vi "4Pi 4Pi Modes - Init DM DUAL.vi"(8 "No hardware":bool=TRUE, 9 "Config File":string, 11 "Base File Path":path) -> (2 "Error out":errorcluster, 3 "DM Handles":T1(array[cluster]))   [LabVIEW 2016]
uses:
  4Pi 4Pi Modes - Controls/4Pi 4Pi Modes - Standard Action.ctl
  Hardware Configuration/Hardware Configuration Controls/Standard Action.ctl
  <userlib>/BMC/BMC.lvlib
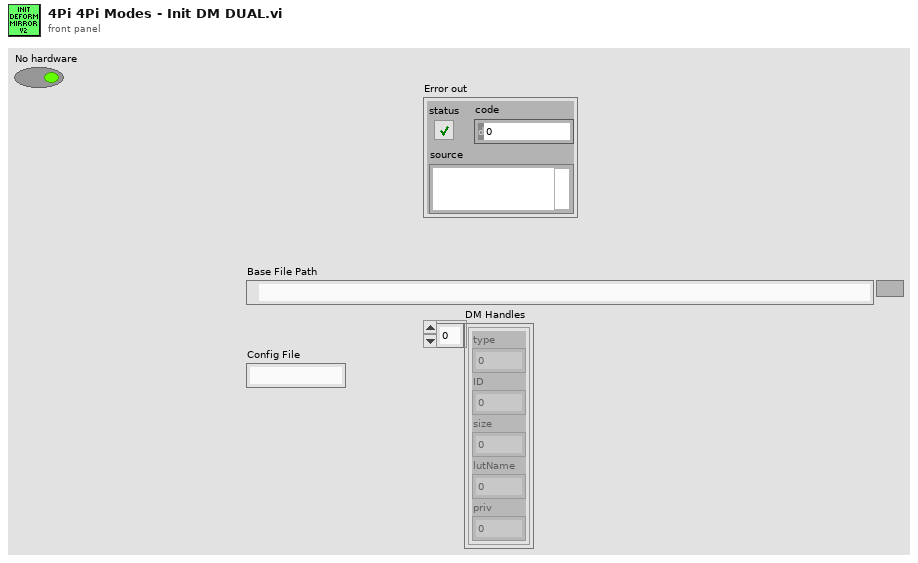
[diagram p1: front panel]
types:
  T1 = cluster{"type":i16, "ID":i16, "size":i32, "lutName":u64, "priv":u64}[]
  T2 = typedef "Standard Action.ctl" = enum16{"Read", "Write"}
  T3 = typedef "4Pi 4Pi Modes - Standard Action.ctl" = enum16{"Read", "Write"}
  T4 = cluster{"Matrix":dbl[][], "Modes":string[], "Flats":dbl[], "Serials":string[]}
  T5 = cluster{"type":i16, "ID":i16, "size":i32, "lutName":u64, "priv":u64}
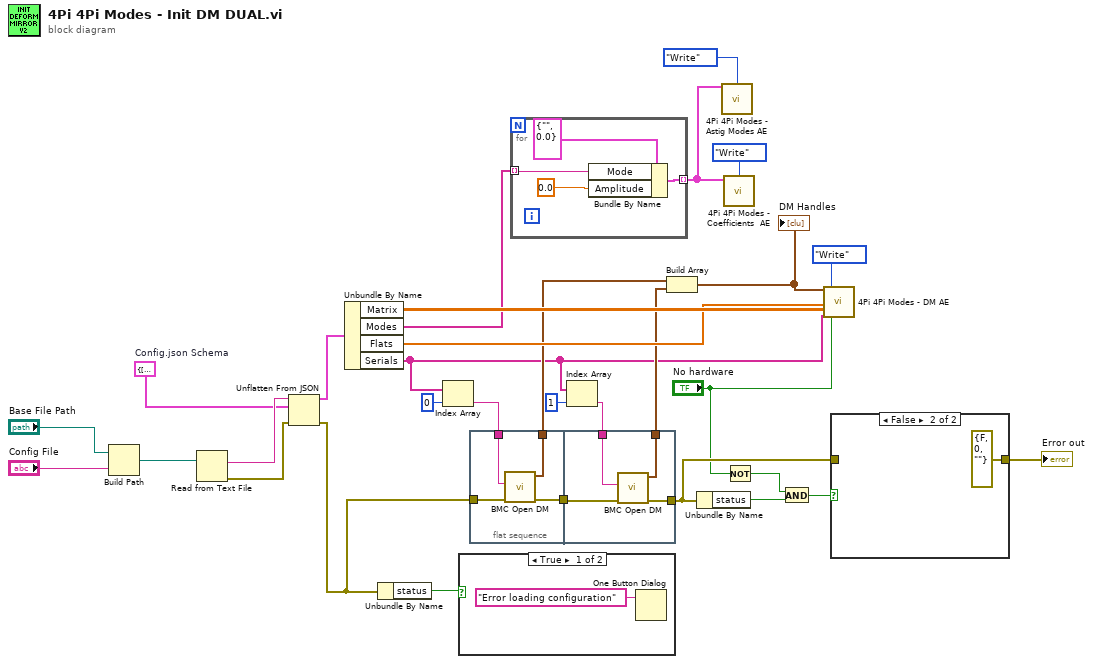
[diagram p0: block diagram]
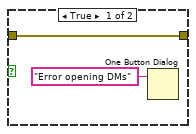
[diagram p2: hidden frame]
diagram:
  w25 = T4 {"Matrix"=[], "Modes"=[], "Flats"=[], "Serials"=[]}  # Config.json Schema
  n1 = Build Path(base path="Base File Path", name or relative path="Config File") -> (appended path=w28:path)
  n2 = Read from Text File(file (use dialog)=w28) -> (text=w26:string, error out=w19:errorcluster)  [unwired: 3 in, 2 out]
  n3 = Unflatten From JSON(JSON string=w26, type and defaults=w25, error in (no error)=w19) -> (value=w24:T4, error out=w18:errorcluster)  [unwired: 4 in]
  n4 = Unbundle By Name(w24) -> ("Matrix"=w23:dbl[][], "Modes"=w9:string[], "Flats"=w22:dbl[], "Serials"=w2:string[])
  n5 = Unbundle By Name(w18) -> ("status"=w27:bool)
  n6 = Index Array(array=w2, index=0) -> (element=w13:string)
  n7 = case shown="True" w27 {
    frame True {
      n8 = One Button Dialog(message="Error loading configuration") -> ()  [unwired: 1 in, 1 out]
    }
    frame False {
    }
  }
  n9 = flat-sequence {
    tunnel: [w36] -> w20
    tunnel: [w35] -> w17
    tunnel: w18 -> [w34]
    tunnel: w13 -> [w33]
    tunnel: w20 -> [w40]
    tunnel: [w39] -> w16
    tunnel: [w38] -> w4
    tunnel: w11 -> [w37]
    frame #0 {
      n10 = call <userlib>:"BMC Open DM.vi"("error in (no error)"=w34, "serial_number"=w33) -> ("error out"=w36:errorcluster, "dmHandle out"=w35:T5)  [unwired: 5 in, 3 out]
    }
    frame #1 {
      n11 = call <userlib>:"BMC Open DM.vi"("error in (no error)"=w40, "serial_number"=w37) -> ("error out"=w38:errorcluster, "dmHandle out"=w39:T5)  [unwired: 5 in, 3 out]
    }
  }
  n12 = for {
    tunnel: w9 -> [w41] mode=indexing
    tunnel: [w43] -> w8 mode=indexing
    n13 = Bundle By Name(cluster=cluster{"Mode":string, "Amplitude":dbl} {"Mode"="", "Amplitude"=0.0}, "Mode"=w41, "Amplitude"=0.0) -> (w43:cluster{"Mode":string, "Amplitude":dbl})
  }
  n14 = Index Array(array=w2, index=1) -> (element=w11:string)
  n15 = Build Array(w17, w16) -> (w15:T1)
  "DM Handles" <- w15
  n16 = Unbundle By Name(w4) -> ("status"=w7:bool)
  n17 = call "4Pi 4Pi Modes - Astig Modes AE.vi"("Coefficients In"=w8, "Action"=Standard_Action."Write") -> ()  [unwired: 12 in, 2 out]
  n18 = call "4Pi 4Pi Modes - Coefficients  AE.vi"("Coefficients In"=w8, "Action"=4Pi_4Pi_Modes_-_Standard_Action."Write") -> ()  [unwired: 13 in, 1 out]
  n19 = Not(x="No hardware") -> (.not. x?=w5:bool)
  n20 = And(x=w5, y=w7) -> (x .and. y?=w6:bool)
  n21 = call "4Pi 4Pi Modes - DM AE.vi"("DM Handles"=w15, "Flats"=w22, "Control Matrix"=w23, "Serials"=w2, "Action"=4Pi_4Pi_Modes_-_Standard_Action."Write", "No hardware"="No hardware") -> ()  [unwired: 9 in, 5 out]
  n22 = case shown="False" w6 {
    tunnel: w4 -> [w45 _]
    tunnel: [w45 errorcluster {"status"=FALSE, "code"=0, "source"=""} ("error out")] -> w3
    frame True {
      n23 = One Button Dialog(message="Error opening DMs") -> ()  [unwired: 1 in, 1 out]
    }
    frame False {
    }
  }
  "Error out" <- w3
